vi "step_12V PS on_off.vi"(8 "error in":errorcluster, 10 "step":T3 {"data num" format="%.3f"}) -> (0 "error out":errorcluster, 2 "test results":T1)   [LabVIEW 2020]
uses:
  controls/PROTO_stepV2.ctl
  controls/step_type.ctl
  controls/test results.ctl
  Hardware Drivers/Keysight E3633 DC PS/dc ps control.ctl
panel:
  in  "test pass":bool
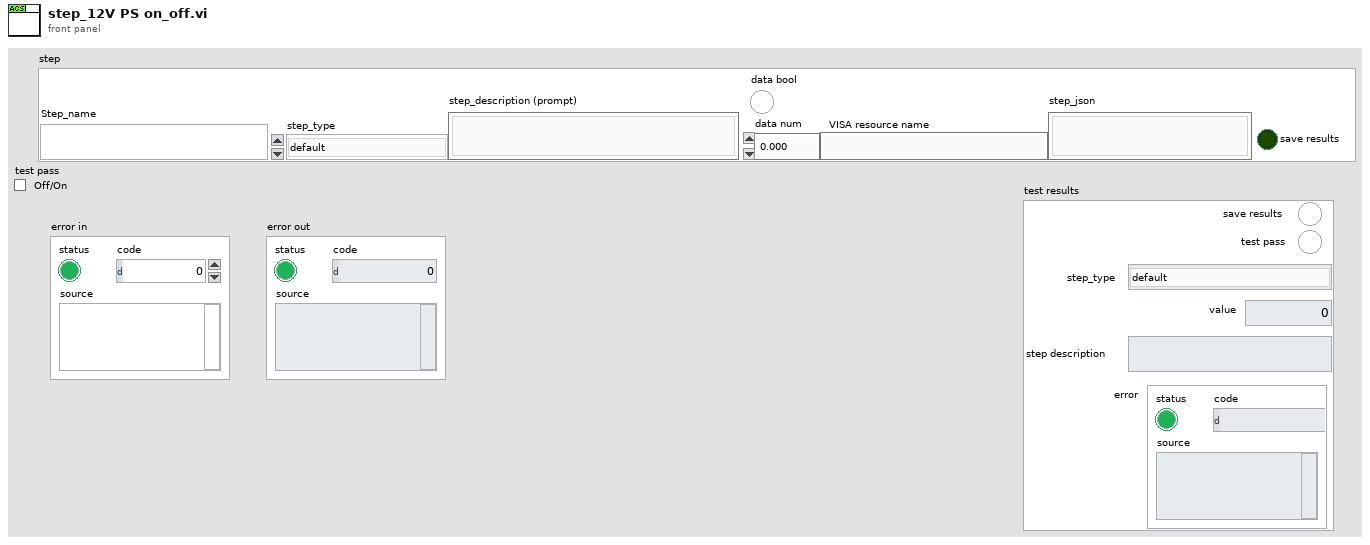
[diagram p1: front panel]
types:
  T1 = typedef "test results.ctl" = cluster{"test pass":bool, "step_type":T2, "value":dbl, "step description":string, "error":errorcluster, "save results":bool}
  T2 = typedef "step_type.ctl" = enum16{"default", "prompt", "sequence#", "12V_1_power supply on_off", "12V_2_power supply on_off", "set_hipot_V", "set_hipot_I_limit", "set_hipot_ramping (sec)", "set hipot_hold_time", "read_hipot_V", "read_hipot_I", "set_daq", "read_daq", "flash uds", "wait (sec)", "record_pass_fail", "ac_charge_test", "dc_400V_charging", "HAPS Heater Output", "HAPS Compressor Output", "stop_test", "error_exit"}
  T3 = typedef "PROTO_stepV2.ctl" = cluster{"VISA resource name":string, "data num":dbl, "step_description (prompt)":string, "step_json":string, "save results":bool, "step_type":T2, "Step_name":string, "data bool":bool}
  T4 = typedef "dc ps control.ctl" = enum16{"init", "config output", "config OVP", "config current limit", "output on_off", "read output", "self test", "close"}
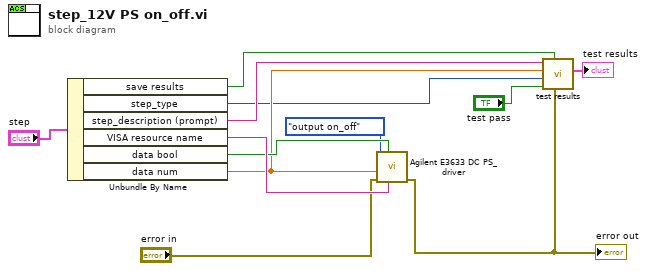
[diagram p0: block diagram]
diagram:
  n1 = Unbundle By Name("step") -> ("save results"=w1:bool, "step_type"=w5:T2, "step_description (prompt)"=w7:string, "VISA resource name"=w12:string, "data bool"=w11:bool, "data num"=w6:dbl)
  n2 = call "Agilent E3633 DC PS_driver.vi"("VISA resource in"=w12, "Enable Output (T: Enable)"=w11, "Error In"="error in", "value in"=w6, "agilent E3633 DC PS"=dc_ps_control."output on_off") -> ("Error Out"=w3:errorcluster)  [unwired: 3 in, 3 out]
  "error out" <- w3
  n3 = call "test results.vi"("error"=w3, "save results"=w1, "test pass"="test pass", "step_type"=w5, "Numeric"=w6, "(description) used in test"=w7) -> ("test results"=→"test results":T1)  [unwired: 5 in]
